vi "Unflatten-QuitEventData.vi"(8 "error in (no error)":errorcluster, 11 "Event Binary Data":string) -> (0 "error out":errorcluster, 3 "Event Data":T1)   [LabVIEW 2026, in "SDL3.lvlib" / "Events.lvlib"]
uses:
  Events.lvlib
  QuitEventData--cluster.ctl
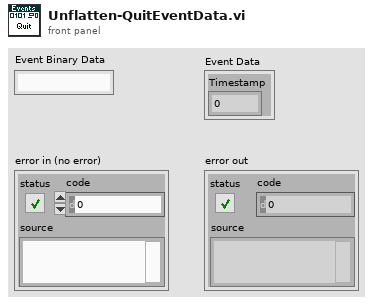
[diagram p1: front panel]
types:
  T1 = typedef "SDL3.lvlib/Events.lvlib/QuitEventData--cluster.ctl" = cluster{"Timestamp":u64}
  T2 = enum16{"big-endian, network order", "native, host order", "little-endian"}
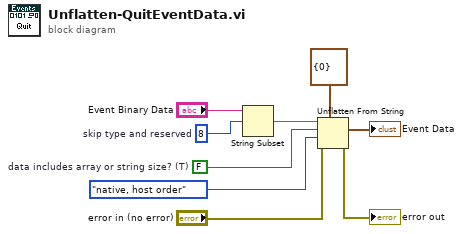
[diagram p0: block diagram]
diagram:
  w3 = 8  # skip type and reserved
  w6 = FALSE  # data includes array or string size? (T)
  n1 = String Subset(string="Event Binary Data", offset (0)=w3) -> (substring=w4:string)  [unwired: 1 in]
  n2 = Unflatten From String(type=T1 {"Timestamp"=0} ("QuitEvent"), binary string=w4, data includes array or string size? (T)=w6, byte order (0:big-endian, network order)=T2."native, host order", error in (no error)="error in (no error)") -> (value=→"Event Data":T1, error out=→"error out":errorcluster)  [unwired: 1 out]
